vi "Stop Core.vi"(10 "final error code":i32, 11 "MC Prompt in":refnum<class "MC Prompt.lvclass">) -> (3 "MC Prompt out":refnum<class "MC Prompt.lvclass">)   [LabVIEW 2024, in "MC Prompt.lvlib" / "MC Prompt.lvclass"]
doc: "<p>(<strong>Filename</strong>: <span class=\"dnl\">Actor Framework.lvlib:Actor.lvclass:Stop Core.vi</span>)</p>\n<p>Defines what the actor does before it stops. Use the <strong>final error code</strong> input to determine whether the actor shut down in response to an error.</p>\n<p>By default, this method passes the Stop message along to all <a href=\"nihelplauncher://docs/csh?context=lvcore_lvcomm_af_launch_nested_actor\">auto-stop nested actors</a>. A descendant class may override this method to define additional behavior, such as shutting down any processes the actor initiated in its override of the <a href=\"nihelplauncher://docs/csh?context=lvcore_lvcomm_af_actor_core\">Actor Core</a> method.</p>"
uses:
  MC Prompt.lvclass
  C:/Program Files/National Instruments/LabVIEW 2024/vi.lib/ActorFramework/Actor/Actor.lvclass
  <vilib>/ActorFramework/Actor/Actor.lvclass/Actor.ctl
  <vilib>/ActorFramework/Message Enqueuer/Message Enqueuer.lvclass/Message Enqueuer.ctl
  <vilib>/ActorFramework/Message Enqueuer/Enqueue.vi
  Controller/Controller Messages/Stop Looking for Buzzer Msg/Stop Looking for Buzzer Msg.lvclass
  C:/Program Files/National Instruments/LabVIEW 2024/vi.lib/ActorFramework/Message/Message.lvclass
  Controller/Controller Messages/Update Player Who Answered Correctly Last Msg/Update Player Who Answered Correctly Last Msg.lvclass
  <vilib>/ActorFramework/Message Priority Queue/Priority Enqueue.vi
  <vilib>/ActorFramework/Actor/Actor.lvclass
  MC Prompt.lvclass/MC Prompt.ctl
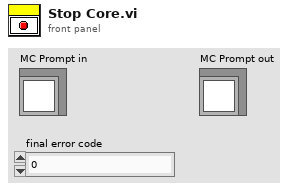
[diagram p1: front panel]
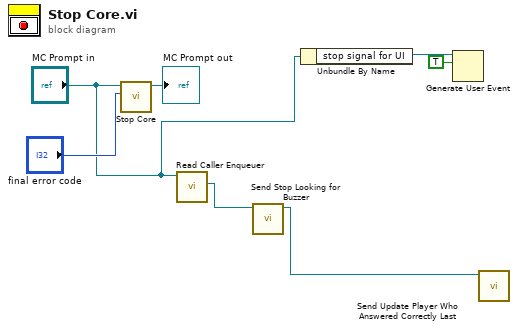
[diagram p0: block diagram]
diagram:
  n1 = call-parent "Stop Core.vi"("final error code"="final error code", "Actor in"="MC Prompt in") -> ("Actor out"=→"MC Prompt out":refnum<class "MC Prompt.lvclass">)  [unwired: 9 in]
  n2 = call <vilib>:"Read Caller Enqueuer.vi"("Actor"="MC Prompt in") -> ("Caller Enqueuer"=w5:refnum<class "Message Enqueuer.lvclass">)  [unwired: 10 in]
  n3 = call "Send Stop Looking for Buzzer.vi"("Message Enqueuer"=w5) -> ("Message Enqueuer out"=w4:refnum<class "Message Enqueuer.lvclass">)  [unwired: 9 in, 1 out]
  n4 = Unbundle By Name("MC Prompt in") -> ("stop signal for UI"=w3:refnum<user-event>)
  n5 = Generate User Event(user event=w3, event data cluster=TRUE ("event data")) -> ()  [unwired: 2 in, 2 out]
  n6 = call "Send Update Player Who Answered Correctly Last.vi"("Message Enqueuer"=w4) -> ()  [unwired: 9 in, 2 out]
